vi "Load.vi"(8 "Error In":errorcluster, 10 "Key":string, 11 "Loader In":refnum<class "Abstract.lvclass">) -> (0 "Error Out":errorcluster, 2 "Template":string, 3 "Loader Out":refnum<class "Abstract.lvclass">)   [LabVIEW 2018, in "Toolkit.lvlib" / "Loaders.lvlib" / "Abstract.lvclass"]
uses:
  Abstract.lvclass
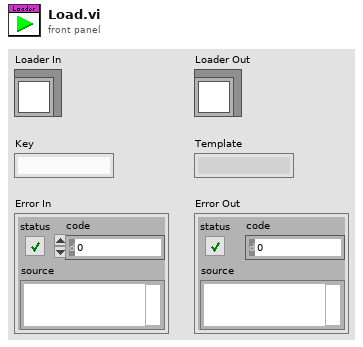
[diagram p1: front panel]
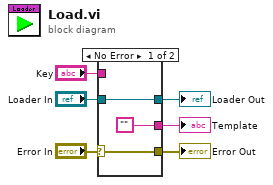
[diagram p0: block diagram]
diagram:
  n1 = case shown="No Error" "Error In" {
    selector: "Error In" -> [w9 w10]
    tunnel: "Loader In" -> [w8 w11]
    tunnel: [w8 w11] -> w5
    tunnel: [w9 w10] -> w3
    tunnel: ["" _] -> w2
    tunnel: "Key" -> [_ _]
    frame No Error {
    }
    frame Error {
    }
  }
  "Loader Out" <- w5
  "Error Out" <- w3
  "Template" <- w2
